vi "Write Digital Port.vi"(8 "error in (no error)":errorcluster, 10 "Relay Mode":bool[](array[boolean]), 11 "DMM in":refnum<class "MIO.lvclass">) -> (0 "error out":errorcluster, 3 "DMM out":refnum<class "MIO.lvclass">)   [LabVIEW 2019, in "Hardware Abstration.lvlib" / "MIO.lvclass"]
uses:
  MIO.lvclass
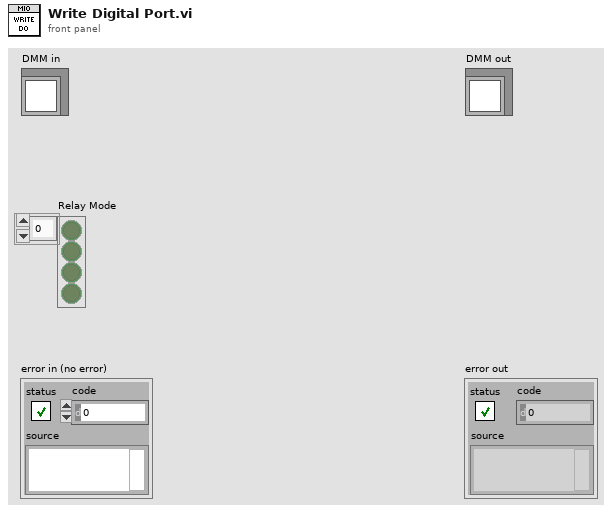
[diagram p1: front panel]
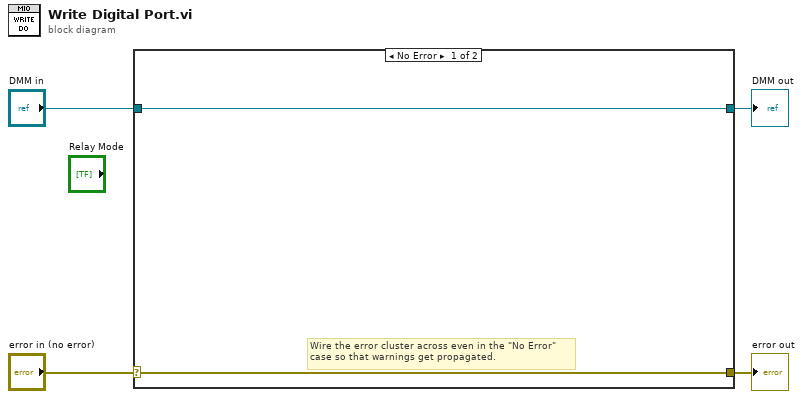
[diagram p0: block diagram]
diagram:
  n1 = case shown="No Error" "error in (no error)" {
    selector: "error in (no error)" -> [w5 w8]
    tunnel: [w5 w8] -> w3
    tunnel: [w6 w7] -> w1
    tunnel: "DMM in" -> [w6 w7]
    frame No Error {
      # "Wire the error cluster across even in the \"No Error\"\ncase so that warnings get propagated."
    }
    frame Error {
    }
  }
  "error out" <- w3
  "DMM out" <- w1
